vi "Globals.vi"() -> ()   [LabVIEW 2013]
panel:
  in  "Rename":string="Renaming Test Cell Controller\n\nPlease be patient, this may take a minute."
  in  "Relative Help Path":string="Help\\Getting Started with the NI Test Cell Control System.pdf"
  in  "Missing Software Error Message":string="The Test Cell Controller software configuration was missing or invalid.  The NI Test Cell Controller software may need to be reinstalled."
  in  "Bad Config Error Message":string="The Test Cell Controller software configuration was missing or invalid.  The NI Test Cell Controller software may need to be reinstalled."
  in  "Relative INI File Path":string="Configuration\\eval_board_config.ini"
  in  "Relative Wiz Path":string="New Test Cell Controller Project.exe"
  in  "Trouble Warning 2":string="Install Failed"
  in  "Product Name":string="cRIO-9082"
  in  "Instructions 2":string="1. Connect the Ethernet cable.\n2. Connect the power cable and press the power button.\n3. Ensure the power LED is on.\n4. Wait 20 seconds for the Test Cell Controller to boot."
  in  "IP Err":string="Go back to Step 2 and check configuration."
  in  "Help URL":string="http://www.ni.com/veristand\""
  in  "IP Trouble Message":string="Failure to detect the Test Cell Controller may be due to one or more of the following:\n\n1. The host computer and Test Cell Controller are on different subnets.\n2. An Ethernet switch or router is off or unplugged.\n3. An Ethernet cable is loose or defective.\n4. The Test Cell Controller was unpowered or booting during the scan.\n\nPlease check for these issues, restart the Test Cell Controller by pressing the reset button, and wait 20 seconds for the Test Cell Controller to boot.\n\nYou can also try setting the IP reset switch to ON, rebooting, waiting 20 seconds, and setting the IP reset switch back to OFF.\n\nTo retry detection, click Rescan for Targets."
  in  "IP Trouble Title":string="Network Troubleshooting Tips"
  in  "Video Path":string="\\Additional Resources\\NIEvalVideo.exe\""
  in  "Success 1":string="Your Test Cell Controller has been successfully configured!\n\nIf you are new to using NI VeriStand, select Launch Getting Started Manual.  Otherwise, select Skip Manual."
  in  "Complete":string="Setup Complete"
  in  "Welcome":string="Welcome to the Test Cell Controller Setup"
  in  "Congrats":string="Congratulations!"
  in  "Restore Time Message":string="Please be patient, this may take several minutes."
  in  "Main Title":string="National Instruments Test Cell Controller Setup"
  in  "Step 5":string="Step 5:\nComplete"
  in  "Step 4":string="Step 4:\nTarget Setup"
  in  "Step 3":string="Step 3:\nHardware Detection"
  in  "Step 2":string="Step 2:\nHardware Setup"
  in  "Step 1":string="Step 1:\nWelcome"
  in  "IMG: Connect Ethernet":string="A. Connect Ethernet and check mode."
  in  "IMG: Connect Power":string="B. Connect power, press power button, and check LED."
  in  "Generic Error Message":string="      Unhandled Error Detected\n\nEnsure the Test Cell Controller is connected properly and reset it.  Then select Previous to retry the operation.  If the operation continues to fail, contact National Instruments for support at (866) 275-6964."
  in  "Manual IP Message":string="Configuring Test Cell Controller IP Address\n\nAttempting Manual IP Assignment..."
  in  "IP Failed":string="Previous Attempt Failed"
  in  "Auto IP":string="Automatic: If your Test Cell Controller is connected to your host PC through an Ethernet switch or router, select Automatic IP to request an IP address via DHCP. Contact your network administrator if your network does not support DHCP."
  in  "Model Code":string="758B"
  in  "Manual IP 1":string="Static (Advanced): If your Test Cell Controller is connected to your host PC directly, enter the appropriate network information below and select Static IP."
  in  "Net Setup":string="Networking Setup and Software Installation\n"
  in  "Reformatting":string="Restoring Test Cell Controller\n\nReformatting ..."
  in  "Reimage Failed Msg":string="Your target did not reimage properly.\nPlease double-check your configuration and then contact support."
  in  "Reimage Success Msg":string="The Test Cell Controller has been successfully restored."
  in  "Reimage Failed":string="Installing Test Cell Controller Software\n\nFailed."
  in  "Reimage Success":string="Installing Test Cell Controller Software\n\nSuccess!"
  in  "Reimaging":string="Installing Test Cell Controller Software\n\nCopying files ..."
  in  "Trouble Warning":string="Restoring the target will erase all existing software on the target and may take several minutes. Please confirm that the MAC address below matches the MAC address printed on the target to be restored.\n\nNote: To be detected after restoration, the target must be located on the same subnet as the host computer."
  in  "Trouble Message":string="1. Please reset the Test Cell Controller (see image below) and wait 20 seconds.\n2. Select Previous, then select Rescan for Targets. \n3. If software install fails multiple times, select Restore Target System to reformat the Test Cell Controller and reimage it with the necessary software. "
  in  "Model Substring":string="RIO"
  in  "Found 2+ Msg":string="1. Check the MAC address of your Test Cell Controller (see image to left for MAC address location).\n2. Verify a MAC address displayed here matches that of your Test Cell Controller.\n3. If a MAC address matches, select it and click Next. \n\nOtherwise, ensure that your hardware is connected properly, then click Rescan for Targets."
  in  "Found 1 Msg":string="1. Check the MAC address of your Test Cell Controller (see image to left for MAC address location).\n2. Verify the MAC address displayed here matches that of your Test Cell Controller.\n\nIf the MAC address matches, click Next.\nOtherwise, ensure your hardware is connected properly, then click Rescan for Targets."
  in  "Found 0 Msg":string="1. Ensure your Test Cell Controller is connected properly.\n2. Restart the Test Cell Controller by pressing the reset button (see image to left for reset button location).\n3. Wait 20 seconds for the Test Cell Controller to boot.\n4.  Click Rescan for Targets.\n\nFor troubleshooting tips, click Troubleshoot."
  in  "Found 2+ Status":string="Detecting Hardware\n\nMultiple Test Cell Controllers detected!"
  in  "Found 1 Status":string="Detecting Hardware\n\nOne Test Cell Controller detected!"
  in  "Found 0 Status":string="Detecting Hardware\n\nNo Test Cell Controllers detected."
  in  "Deployment Finished":string="Testing Configuration\n\nTarget software is configured correctly"
  in  "DHCP Message":string="Configuring Test Cell Controller IP Address\n\nAttempting Automatic IP Assignment..."
  in  "Deployment Message":string="Software Install Required\n\nSelect Begin Install to install to the target."
  in  "Success 2":string="1. Please record the Test Cell Controller's IP Address (displayed above). It is needed for use in NI VeriStand.\n2. Click Exit Setup and Launch New Project Wizard to create a new Test Cell Controller Project."
  in  "Deployment in Progress":string="Software Install\n\nInstalling to Test Cell Controller..."
  in  "Detecting in Progress":string="Detecting Hardware\n\nSearching for Test Cell Controllers..."
  in  "Detection Message":string="Click the button below to find the hardware you just connected."
  in  "Instructions Title":string="Connect Your Test Cell Controller Hardware"
  in  "Welcome Message":string="This wizard helps to ensure that your hardware is connected and configured properly to be used as a target in a NI VeriStand system definition.\n\n\nNote: During setup and also during the tutorials, your firewall software may prompt you to block or unblock the National Instruments software.  Select unblock whenever you encounter this prompt."
  # "OR"
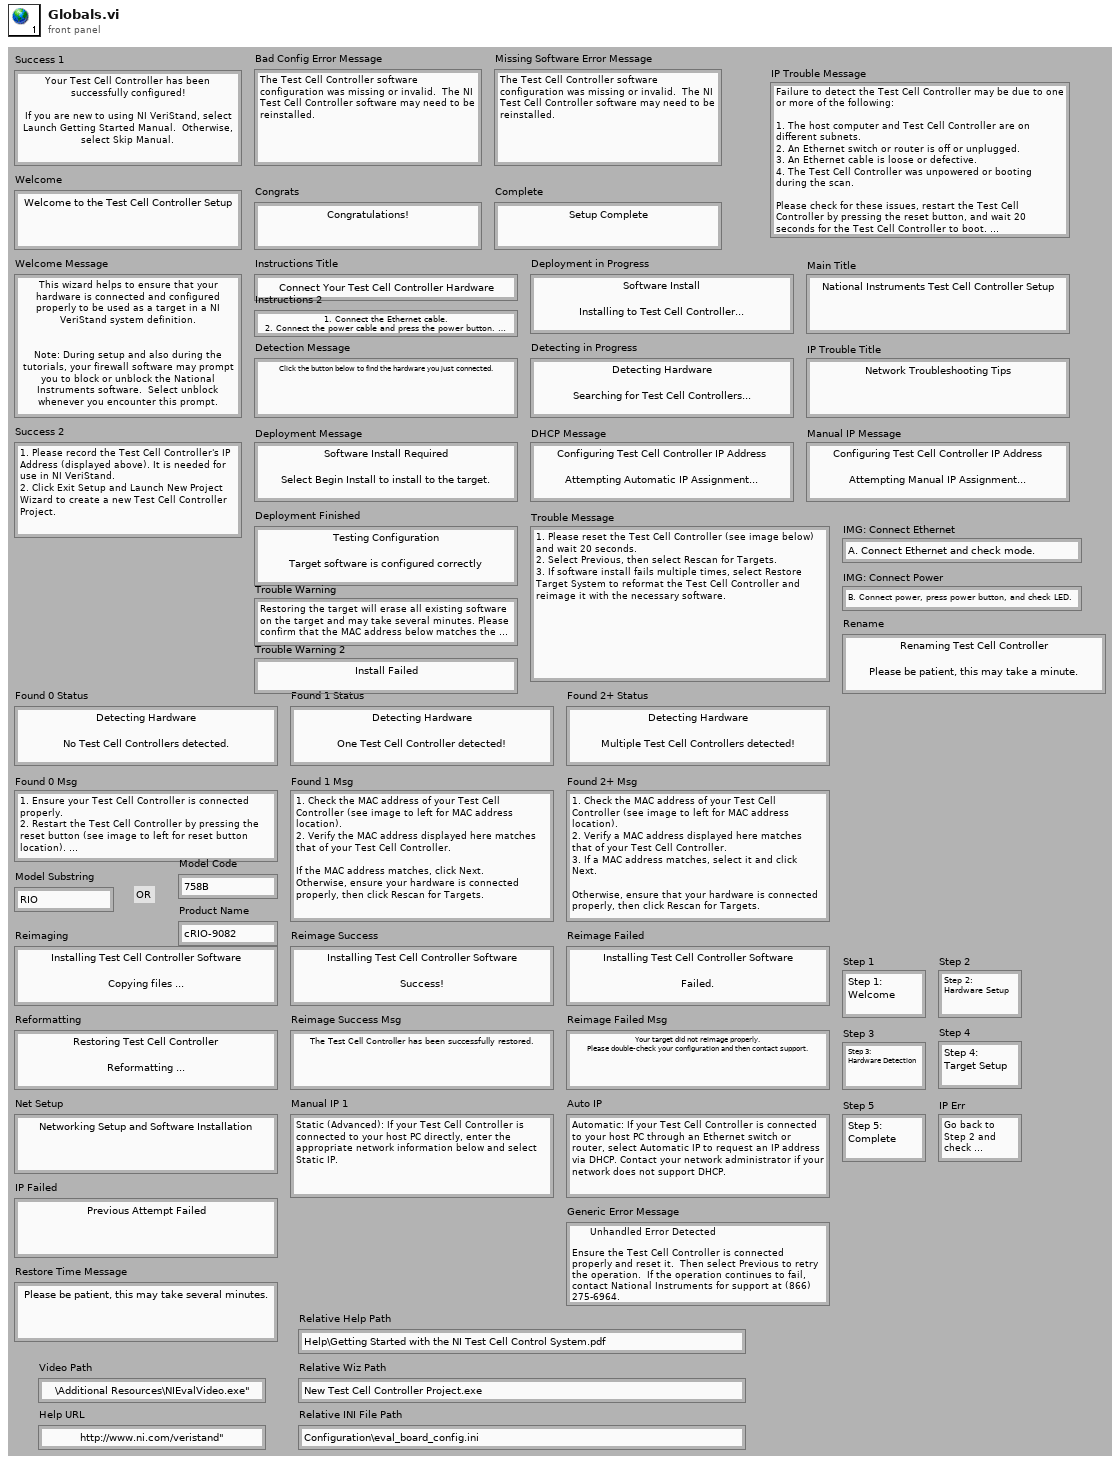
[diagram p1: front panel]
diagram:
